vi "protect_EOL_symbols.vi"(8 "error in (no error)":errorcluster, 11 "String":string) -> (0 "error out":errorcluster, 3 "result string":string)   [LabVIEW 2015, in "ini_work_Library.lvlib"]
doc: "Replaces all EOL to /n forcorrect save in ini file"
uses:
  ini_work_Library.lvlib
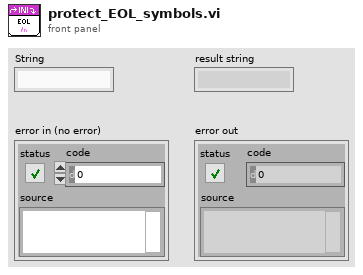
[diagram p1: front panel]
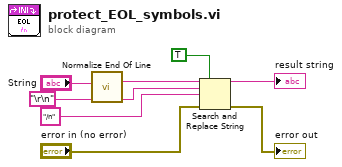
[diagram p0: block diagram]
diagram:
  n1 = call <vilib>:"Normalize End Of Line.vi"("string in"="String") -> ("string out"=w3:string)  [unwired: 7 in]
  n2 = Search and Replace String(replace all?=TRUE ("replace all? (F)"), input string=w3, search string="\r\n", replace string="/n" ("replace string (\"\")"), error in="error in (no error)") -> (result string=→"result string":string, error out=→"error out":errorcluster)  [unwired: 3 in, 2 out]
